vi "Get AI param from DB.vi"(4 "password":string, 6 "connection information":path=path "C:/temp/H1.udl", 7 "KFM":string[](array[string]), 8 "error in (no error)":errorcluster, 9 "AIParamColumns":string[](array[string])=["instrument_gain", "instrument_offset", "time_const", "instrument_min_offset", "instrument_range_min", "process_range_min", "process_low_acd", "process_low_alr", "process_high_alr", "process_high_acd", "process_range_max", "instrument_range_max", "instrument_max_offset", "d", "input_register_min", "input_register_max", "input_pv_min", "input_pv_max", "module_fcode_full", "control_channel_num", "ip_adress", "fcode", "fcodef", "fcode_full", "fname", "process_units"], 10 "AIParamTable":string="fa_3", 11 "AIParameters":string[](array[string])) -> (0 "error out":errorcluster, 2 "Names table":string[][](array[string]), 3 "Parameters table":dbl[][](array[numeric]))   [LabVIEW 2019, in "Inputs.lvlib"]
uses:
  Inputs.lvlib
  <vilib>/addons/database/Connection.llb/DB Tools Open Connec (Path).vi
  Database/Progress.vi
  <vilib>/addons/database/_DB Variant To Data/Database Variant To Data.xnode
  Database/PostgreSQL.lvlib
  <vilib>/addons/database/NI_Database_API.lvlib
panel:
  # "fcode_full"
  # "fname"
  # "process_unit"
  # "time_const"
  # "instrument_min_offset"
  # "process_range_min"
  # "process_low_acd"
  # "instrument_range_max"
  # "d"
  # "input_register_min"
  # "input_register_max"
  # "input_pv_min"
  # "input_pv_max"
  # "ip_adress"
  # "fcodef"
  # "instrument_max_offset"
  # "instrument_range_min"
  # "control_channel_num"
  # "process_range_max"
  # "instrument_offset"
  # "process_high_acd"
  # "process_high_alr"
  # "instrument_gain"
  # "process_low_alr"
  # "module_num"
  # "fcode"
  # "Names"
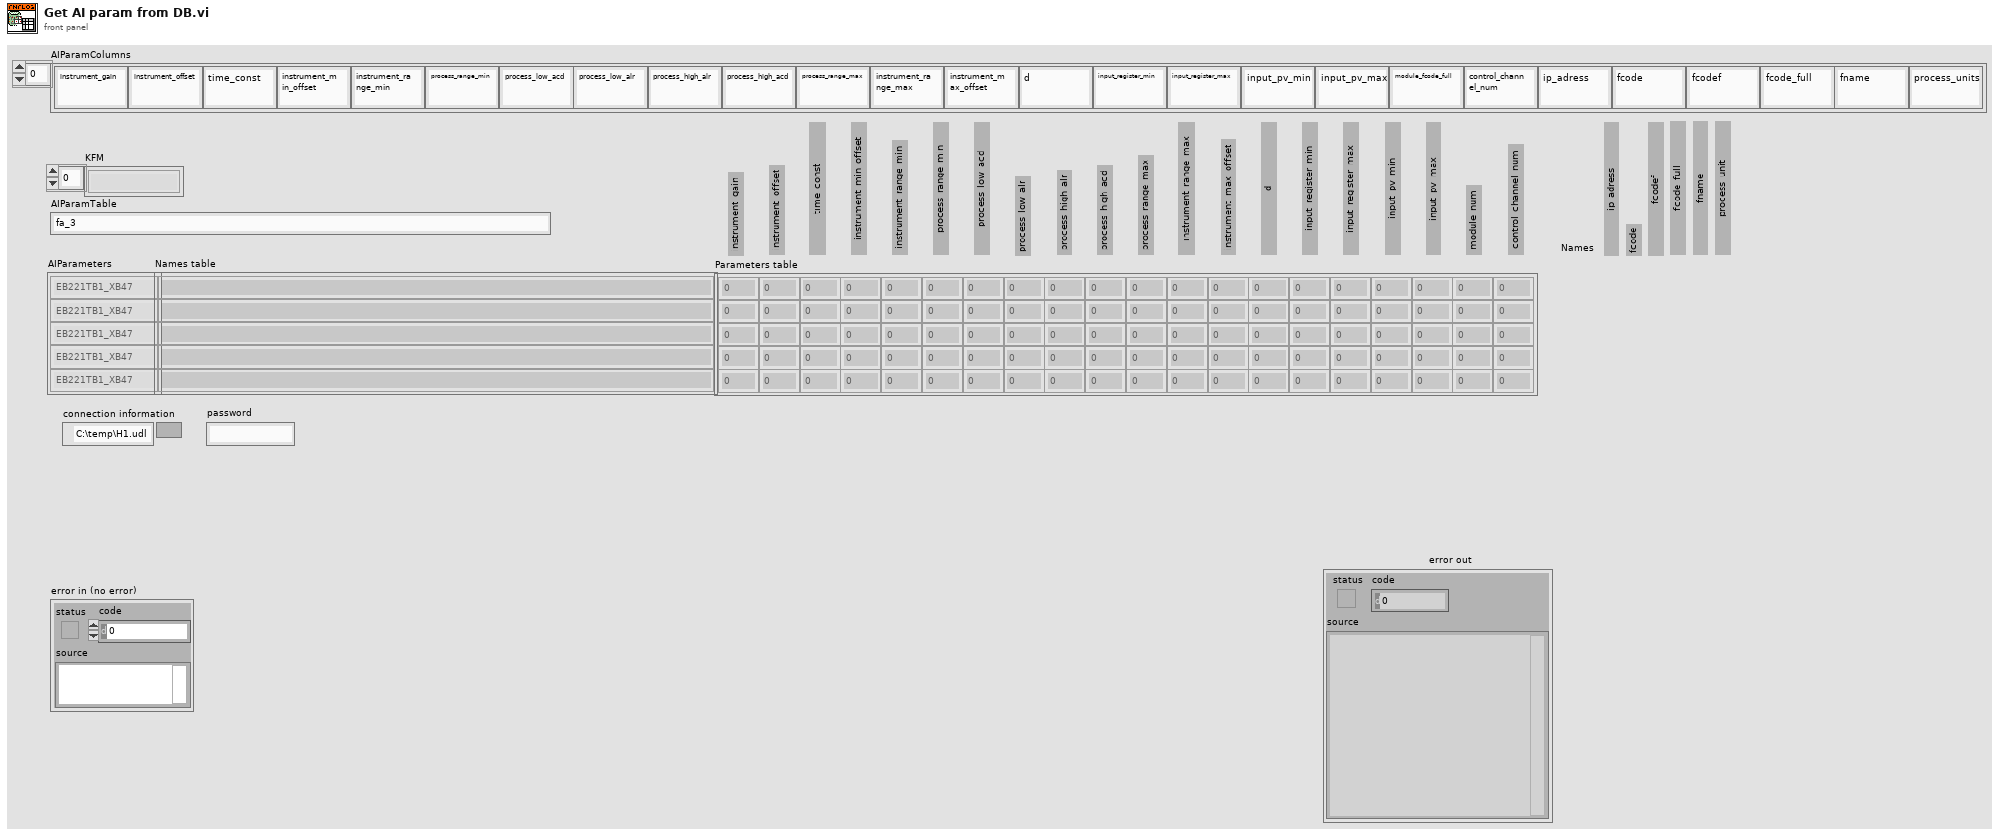
[diagram p1: front panel]
types:
  T1 = typedef "NI_Database_API.lvlib/Conn ObjectReference.ctl" = refnum<k1>
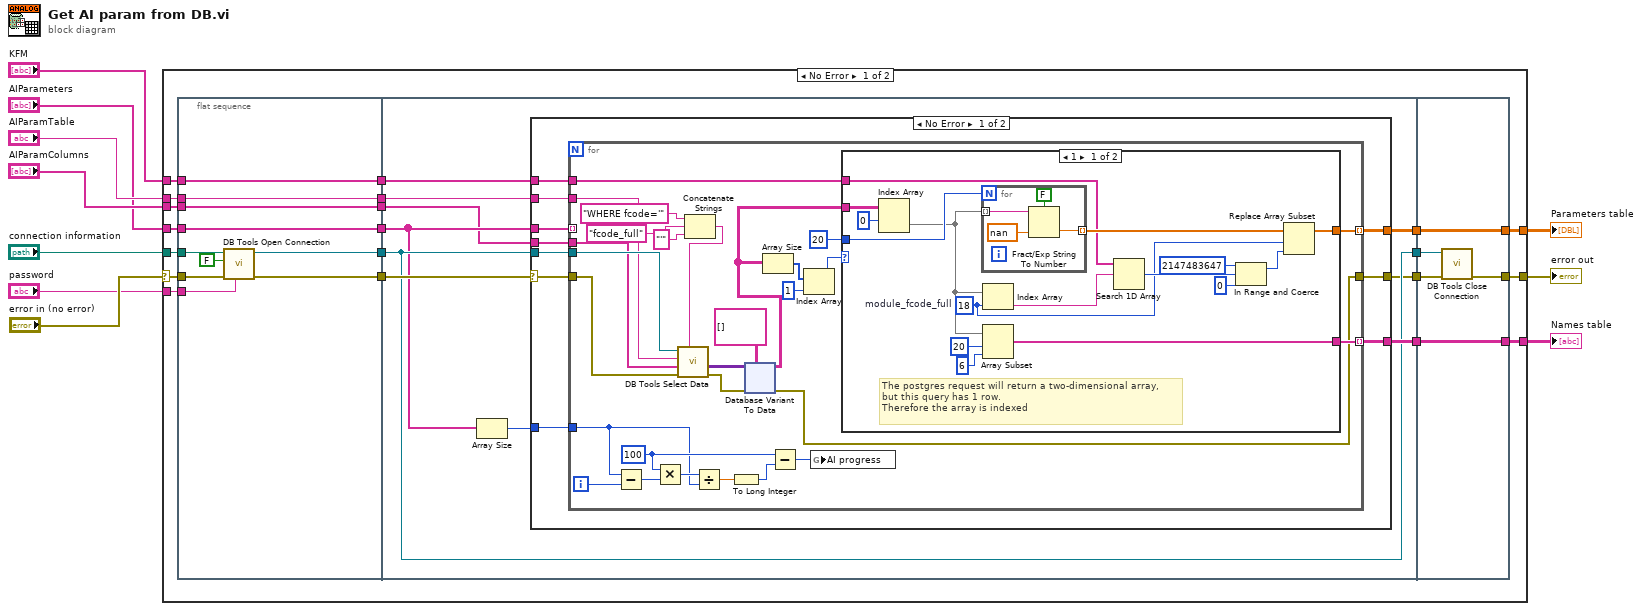
[diagram p0: block diagram]
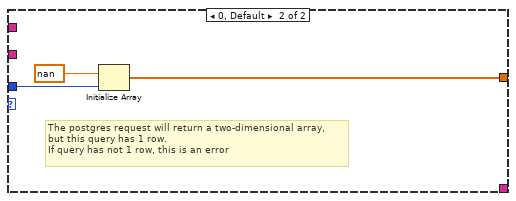
[diagram p2: hidden frame]
diagram:
  n1 = case shown="No Error" "error in (no error)" {
    selector: "error in (no error)" -> [w14 w162]
    tunnel: [w21 w162] -> w10
    tunnel: [w20 _] -> w9
    tunnel: [w19 _] -> w8
    tunnel: "AIParamColumns" -> [w18 _]
    tunnel: "connection information" -> [w17 _]
    tunnel: "AIParamTable" -> [w16 _]
    tunnel: "AIParameters" -> [w15 _]
    tunnel: "KFM" -> [w13 _]
    tunnel: "password" -> [w11 _]
    frame No Error {
      n2 = flat-sequence {
        tunnel: [w40] -> w30
        tunnel: [w39] -> w29
        tunnel: [w32] -> w28
        tunnel: w15 -> [w38]
        tunnel: w16 -> [w40]
        tunnel: w18 -> [w39]
        tunnel: w17 -> [w35]
        tunnel: [w31] -> w27
        tunnel: [w38] -> w26
        tunnel: w14 -> [w33]
        tunnel: w13 -> [w37]
        tunnel: [w37] -> w12
        tunnel: w11 -> [w34]
        tunnel: w30 -> [w42]
        tunnel: w29 -> [w41]
        tunnel: w28 -> [w47]
        tunnel: [w50] -> w25
        tunnel: [w49] -> w24
        tunnel: w27 -> [w46]
        tunnel: w26 -> [w45]
        tunnel: [w46] -> w23
        tunnel: [w44] -> w22
        tunnel: w12 -> [w43]
        tunnel: [w161] -> w20
        tunnel: w25 -> [w161]
        tunnel: [w157] -> w21
        tunnel: w24 -> [w160]
        tunnel: [w160] -> w19
        tunnel: w23 -> [w159]
        tunnel: w22 -> [w158]
        frame #0 {
          n3 = call-poly <vilib>:"DB Tools Open Connection.vi"("password"=w34, "error in (no error)"=w33, "prompt? (F)"=FALSE, "connection information"=w35) -> ("error out"=w32:errorcluster, "connection reference"=w31:T1)  [unwired: 4 in]
        }
        frame #1 {
          n4 = Array Size(array=w45) -> (size(s)=w48:i32)
          n5 = case shown="No Error" w47 {
            selector: w47 -> [w58 w156]
            tunnel: w45 -> [w56 _]
            tunnel: [w60 _] -> w50
            tunnel: [w59 _] -> w49
            tunnel: w48 -> [w57 _]
            tunnel: w46 -> [w55 _]
            tunnel: w42 -> [w54 _]
            tunnel: [w53 w156] -> w44
            tunnel: w43 -> [w52 _]
            tunnel: w41 -> [w51 _]
            frame No Error {
              n6 = for {
                tunnel: [w88] -> w59 mode=indexing
                tunnel: [w87] -> w60 mode=indexing
                tunnel: w58 -> [w72]
                tunnel: w57 -> [w79]
                tunnel: w56 -> [_] mode=indexing
                tunnel: w55 -> [w73]
                tunnel: w54 -> [w71]
                tunnel: [w66] -> w53
                tunnel: w52 -> [w77]
                tunnel: w51 -> [w67]
                i -> [w80]
                w84 = 100 ("y")
                n7 = Subtract(x=w79, y=w80) -> (x-y=w83:i32)
                n8 = Multiply(x=w84, y=w83) -> (x*y=w86:i32)
                n9 = Concatenate Strings("WHERE fcode='" ("table"), "fcode_full" ("Column name"), "'" ("table")) -> (w68:string)
                n10 = call <vilib>:"DB Tools Select Data.vi"("condition"=w68, "error in (no error)"=w72, "columns"=w67, "table"=w71, "connection reference"=w73) -> ("error out"=w76:errorcluster, "data"=w75:variant[][])  [unwired: 1 in, 1 out]
                n11 = Divide(x=w86, y=w79) -> (x/y=w82:dbl)
                n12 = To Long Integer(number=w82) -> (32bit integer=w81:i32)
                n13 = xnode "Database Variant To Data"("database variant"=w75, "error in (no error)"=w76, "type"=string[][] [] ("columns")) -> ("data"=w65:string[][], "error out"=w66:errorcluster)
                n14 = Array Size(array=w65) -> (size(s)=w64:i32[])
                n15 = Subtract(x=w84, y=w81) -> (x-y=w85:i32)
                n16 = Index Array(array=w64, index=1) -> (element=w62:i32)
                n17 = global write "Progress.vi" "AI progress"(w85) -> ()
                n18 = case shown="1" w62 {
                  tunnel: [w138 w154] -> w87
                  tunnel: u32 20 ("y") -> [w143 w153]
                  tunnel: w65 -> [w142 _]
                  tunnel: [w145 _] -> w88
                  tunnel: w77 -> [w140 _]
                  frame 1 {
                    w133 = 18  # module_fcode_full
                    # "The postgres request will return a two-dimensional array,\nbut this query has 1 row.\nTherefore the array is indexed"
                    n19 = Index Array(array=w142, index (row)=0) -> (element=w141:string[])  [unwired: 1 in]
                    n20 = for {
                      N: w143 -> [_]
                      tunnel: w141 -> [w151] mode=indexing
                      tunnel: [w150] -> w148 mode=indexing
                      n21 = Fract/Exp String To Number(use system decimal point (T)=FALSE, string=w151, default (0 dbl)=nan) -> (number=w150:dbl)  [unwired: 1 in, 1 out]
                    }
                    n22 = Index Array(array=w141, index=w133) -> (element=w139:string)
                    n23 = Array Subset(array=w141, index=20, length=6) -> (w145:string[])
                    n24 = Search 1D Array(1D array=w140, element=w139) -> (index of element=w137:i32)  [unwired: 1 in]
                    n25 = In Range and Coerce(upper limit=2147483647, x=w137, lower limit=0) -> (coerced(x)=w134:i32)  [unwired: 1 out]
                    n26 = Replace Array Subset(array=w148, new element=w134, index=w133) -> (w138:dbl[])
                  }
                  frame 0, Default {
                    # "The postgres request will return a two-dimensional array,\nbut this query has 1 row.\nIf query has not 1 row, this is an error"
                    n27 = Initialize Array(nan, w153) -> (w154:dbl[])
                  }
                }
              }
            }
            frame Error {
            }
          }
        }
        frame #2 {
          n28 = call <vilib>:"DB Tools Close Connection.vi"("error in (no error)"=w158, "connection reference"=w159) -> ("error out"=w157:errorcluster)  [unwired: 5 in]
        }
      }
    }
    frame Error {
    }
  }
  "error out" <- w10
  "Parameters table" <- w9
  "Names table" <- w8
